vi "ConfigRange.vi"(0 "VISA resource name":refnum<visa-resource-name>, 1 "Range":T1(ring), 3 "error in (no error)":errorcluster) -> (7 "VISA resource name out":refnum<visa-resource-name>, 10 "error out":errorcluster)   [LabVIEW 2016]
panel:
  in  "Frequency (1:1kHz)":u16(ring)=1 items=["120 Hz Frequency", "1 kHz Frequency", "1 MHz Frequency"]
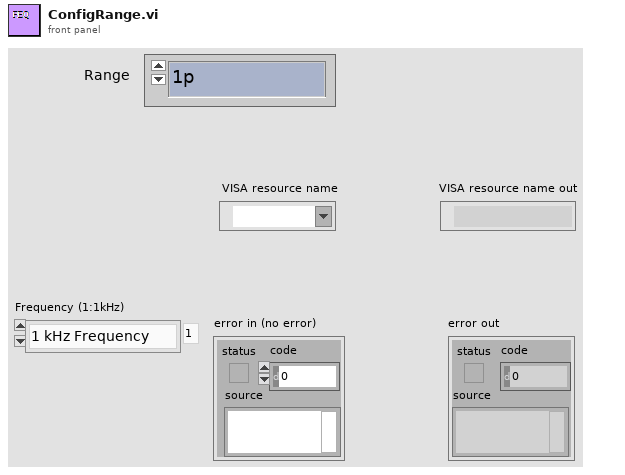
[diagram p1: front panel]
types:
  T1 = enum16{"1p", "2.2p", "4.7p", "10p", "22p", "47p", "100p", "220p", "470p", "1n", "2.2n", "4.7n", "10n", "22n", "47n", "100n", "220n", "470n", "1u", "2.2u", "4.7u", "10u", "22u", "47u", "100u", "220u", "470u", "1m", "AUTO", ""}
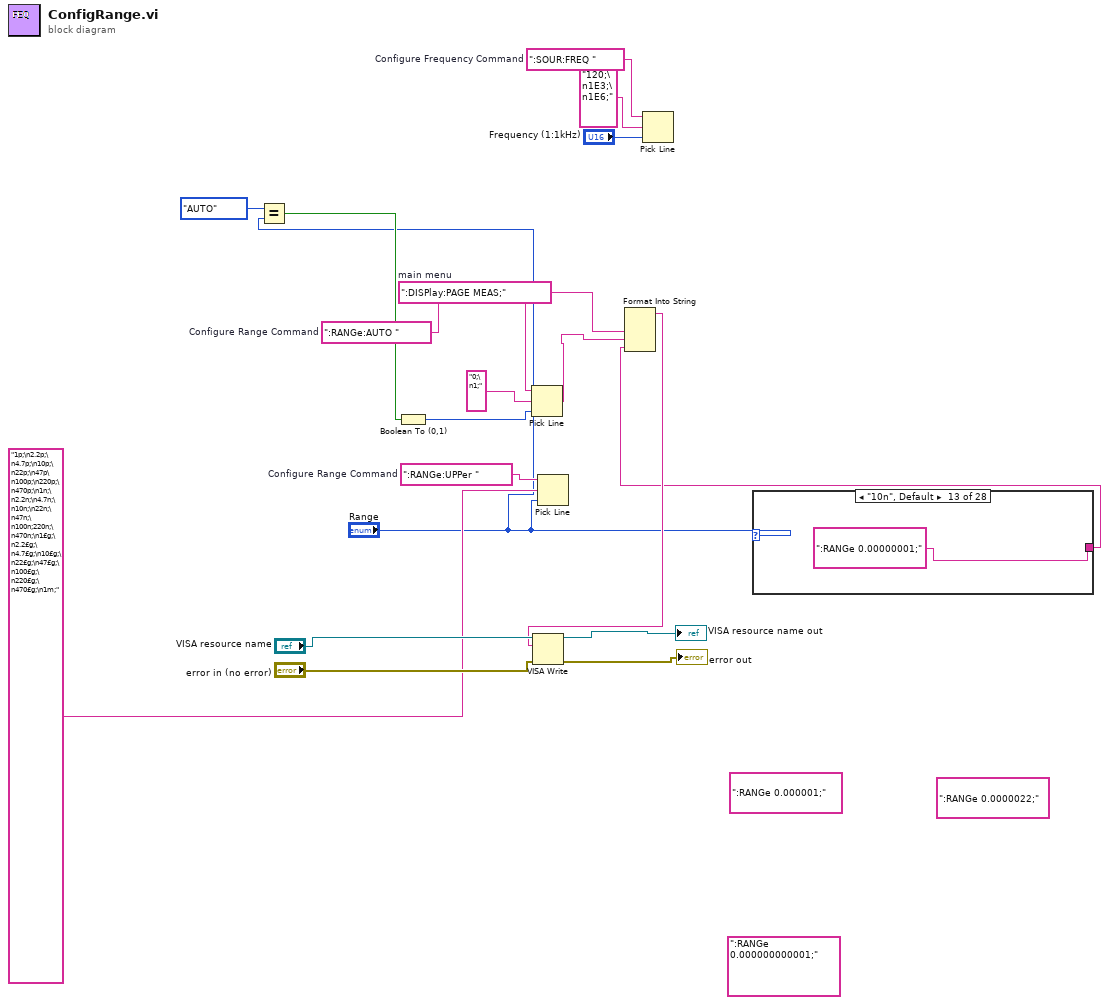
[diagram p0: block diagram]
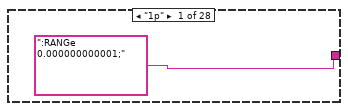
[diagram p2: hidden frame]
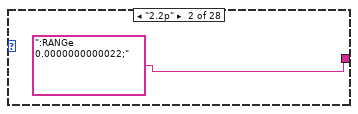
[diagram p3: hidden frame]
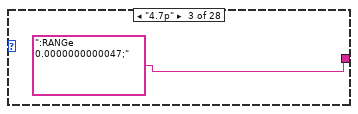
[diagram p4: hidden frame]
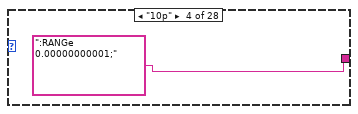
[diagram p5: hidden frame]
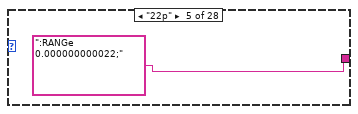
[diagram p6: hidden frame]
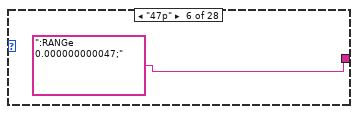
[diagram p7: hidden frame]
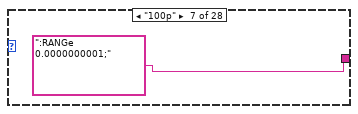
[diagram p8: hidden frame]
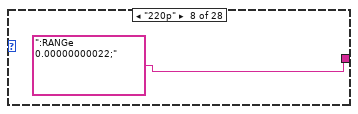
[diagram p9: hidden frame]
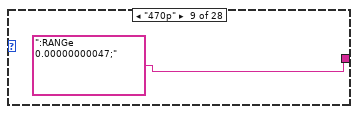
[diagram p10: hidden frame]
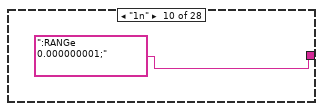
[diagram p11: hidden frame]
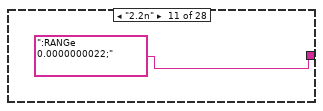
[diagram p12: hidden frame]
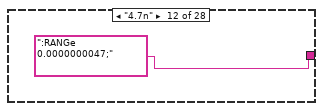
[diagram p13: hidden frame]
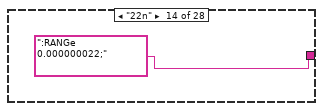
[diagram p14: hidden frame]
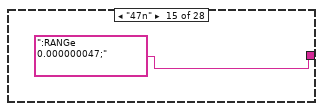
[diagram p15: hidden frame]
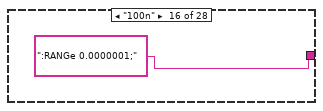
[diagram p16: hidden frame]
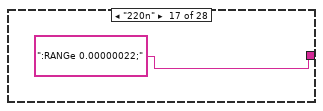
[diagram p17: hidden frame]
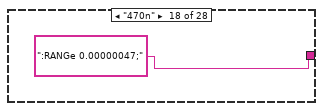
[diagram p18: hidden frame]
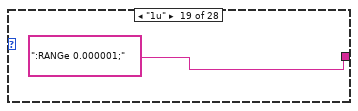
[diagram p19: hidden frame]
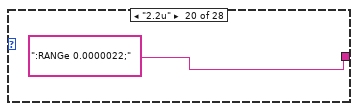
[diagram p20: hidden frame]
diagram:
  (unwired) ":RANGe 0.0000022;" ("Configure Range Command")
  (unwired) ":RANGe 0.000000000001;" ("Configure Range Command")
  (unwired) ":RANGe 0.000001;" ("Configure Range Command")
  w10 = ":RANGe:UPPer "  # Configure Range Command
  w7 = ":RANGe:AUTO "  # Configure Range Command
  w14 = ":DISPlay:PAGE MEAS;"  # main menu
  w17 = ":SOUR:FREQ "  # Configure Frequency Command
  n1 = Equal?(x=T1."AUTO", y="Range") -> (x = y?=w5:bool)
  n2 = Boolean To (0,1)(Boolean=w5) -> (0, 1=w4:i16)
  n3 = Pick Line(string ("")=w7, multi-line string="0;\n1;", line index=w4) -> (output string=w3:string)
  n4 = Pick Line(string ("")=w10, multi-line string="1p;\n2.2p;\n4.7p;\n10p;\n22p;\n47p\n100p;\n220p;\n470p;\n1n;\n2.2n;\n4.7n;\n10n;\n22n;\n47n;\n100n;220n;\n470n;\n1£g;\n2.2£g;\n4.7£g;\n10£g;\n22£g;\n47£g;\n100£g;\n220£g;\n470£g;\n1m;", line index="Range") -> ()  [unwired: 1 out]
  n5 = Pick Line(string ("")=w17, multi-line string="120;\n1E3;\n1E6;", line index="Frequency (1:1kHz)") -> ()  [unwired: 1 out]
  n6 = case shown="\"10n\", Default" "Range" {
    tunnel: [":RANGe 0.000000000001;" ("Configure Range Command") ":RANGe 0.0000000000022;" ("Configure Range Command") ":RANGe 0.0000000000047;" ("Configure Range Command") ":RANGe 0.00000000001;" ("Configure Range Command") ":RANGe 0.000000000022;" ("Configure Range Command") ":RANGe 0.000000000047;" ("Configure Range Command") ":RANGe 0.0000000001;" ("Configure Range Command") ":RANGe 0.00000000022;" ("Configure Range Command") ":RANGe 0.00000000047;" ("Configure Range Command") ":RANGe 0.000000001;" ("Configure Range Command") ":RANGe 0.0000000022;" ("Configure Range Command") ":RANGe 0.0000000047;" ("Configure Range Command") ":RANGe 0.00000001;" ("Configure Range Command") ":RANGe 0.000000022;" ("Configure Range Command") ":RANGe 0.000000047;" ("Configure Range Command") ":RANGe 0.0000001;" ("Configure Range Command") ":RANGe 0.00000022;" ("Configure Range Command") ":RANGe 0.00000047;" ("Configure Range Command") ":RANGe 0.000001;" ("Configure Range Command") ":RANGe 0.0000022;" ("Configure Range Command") ":RANGe 0.0000047;" ("Configure Range Command") ":RANGe 0.00001;" ("Configure Range Command") ":RANGe 0.000022;" ("Configure Range Command") ":RANGe 0.000047;" ("Configure Range Command") ":RANGe 0.0001;" ("Configure Range Command") ":RANGe 0.00022;" ("Configure Range Command") ":RANGe 0.00047;" ("Configure Range Command") ":RANGe 0.001;" ("Configure Range Command")] -> w1
    frame "1p" {
    }
    frame "2.2p" {
    }
    frame "4.7p" {
    }
    frame "10p" {
    }
    frame "22p" {
    }
    frame "47p" {
    }
    frame "100p" {
    }
    frame "220p" {
    }
    frame "470p" {
    }
    frame "1n" {
    }
    frame "2.2n" {
    }
    frame "4.7n" {
    }
    frame "10n", Default {
    }
    frame "22n" {
    }
    frame "47n" {
    }
    frame "100n" {
    }
    frame "220n" {
    }
    frame "470n" {
    }
    frame "1u" {
    }
    frame "2.2u" {
    }
    frame "4.7u" {
    }
    frame "10u" {
    }
    frame "22u" {
    }
    frame "47u" {
    }
    frame "100u" {
    }
    frame "220u" {
    }
    frame "470u" {
    }
    frame "1m" {
    }
  }
  n7 = Format Into String(w14, w3, w1) -> (resulting string=w11:string)  [unwired: 3 in, 1 out]
  n8 = VISA Write(VISA resource name="VISA resource name", write buffer=w11, error in (no error)="error in (no error)") -> (VISA resource name out=→"VISA resource name out":refnum<visa-resource-name>, error out=→"error out":errorcluster)  [unwired: 1 out]
